vi "Filter Predicate.vi"(10 "Filter":T1, 11 "Status":T2) -> (3 "Include?":bool)   [LabVIEW 2020, in "Result Model.lvclass"]
uses:
  Result Model.lvclass
  Result/Status.ctl
  Tree Item Filter.ctl
  Result/Result.lvlib
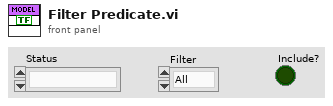
[diagram p1: front panel]
types:
  T1 = typedef "Result Model.lvclass/Tree Item Filter.ctl" = enum16{"All", "Only Fails"}
  T2 = typedef "Result.lvlib/Status.ctl" = enum16{"", "Passed", "Failed", "Error", "Skipped", "Setup Error", "Broken", "Teardown Error"}
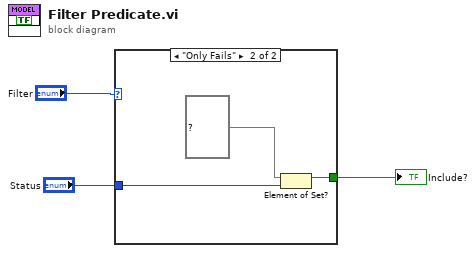
[diagram p0: block diagram]
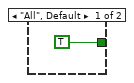
[diagram p2: hidden frame]
diagram:
  n1 = case shown="\"Only Fails\"" "Filter" {
    tunnel: "Status" -> [_ w7]
    tunnel: [TRUE w6] -> w1
    frame "All", Default {
    }
    frame "Only Fails" {
      n2 = Element of Set?(10:w7, 11:set{T2} {enum."", enum."Failed", enum."Error", enum."Setup Error", enum."Broken", enum."Teardown Error"} ("set out")) -> (3:w6:bool)
    }
  }
  "Include?" <- w1
